vi "set_change_value.vi"(0 "数值输入":dbl, 1 "step5":dbl, 2 "Turning Point1":dbl, 3 "step4":dbl, 4 "step1":dbl, 6 "Turning Point4":dbl, 7 "step2":dbl, 8 "Desitination Value":dbl, 9 "Turning Point2":dbl, 10 "精度":dbl, 11 "step3":dbl, 13 "Turing Pont3":dbl) -> (14 "数值输出":sgl)   [LabVIEW 2014]
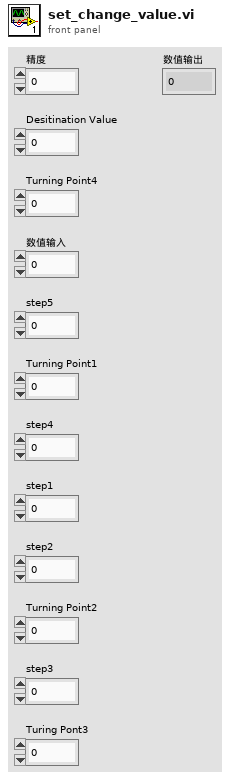
[diagram p1: front panel]
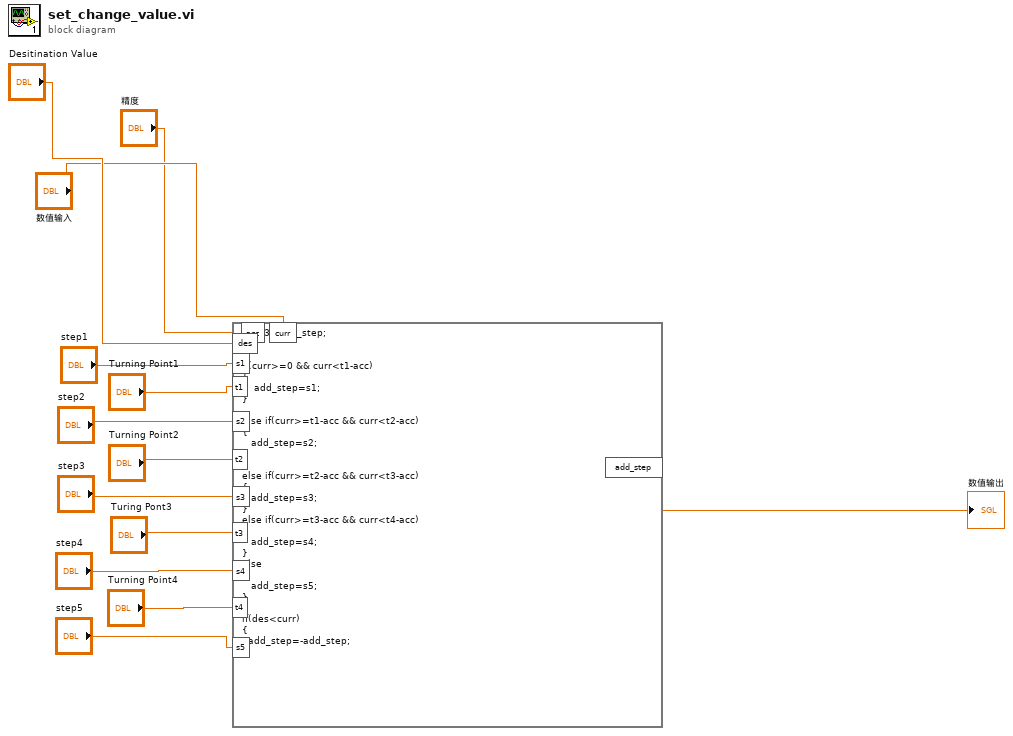
[diagram p0: block diagram]
diagram:
  n1 = formula code="float32 add_step;\n\n\nif(curr>=0 && curr<t1-acc)\n{\n    add_step=s1;\n}\n\nelse if(curr>=t1-acc && curr<t2-acc)\n{\n   add_step=s2;\n}\n\nelse if(curr>=t2-acc && curr<t3-acc)\n{\n   add_step=s3;\n}\nelse if(curr>=t3-acc && curr<t4-acc)\n{\n   add_step=s4;\n}\nelse\n{\n   add_step=s5;\n}\n\nif(des<curr)\n{\n  add_step=-add_step;\n}"("t1"="Turning Point1", "s2"="step2", "t2"="Turning Point2", "s3"="step3", "t3"="Turing Pont3", "s4"="step4", "t4"="Turning Point4", "s5"="step5", "s1"="step1", "acc"="精度", "curr"="数值输入", "des"="Desitination Value") -> ("add_step"=→"数值输出":sgl)
